vi "control 2.vi"() -> ()   [LabVIEW 2010]
uses:
  <vilib>/Analysis/NI_AALBase.lvlib
panel:
  in  "Ajuste ON?":bool=TRUE
  in  "Control ON?":bool=TRUE
  in  "N Prom":i32
  in  "N Prom inicial":i32
  in  "dSigma":dbl
  in  "dAmp":dbl
  in  "dt0":dbl
  in  "SigmaMax":dbl
  in  "time (ms)":dbl
  in  "# samples":i32
  in  "AmpMax":dbl
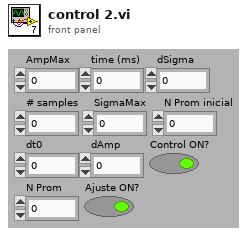
[diagram p1: front panel]
types:
  T1 = cluster{"Amplitud":dbl, "Media":dbl, "Sigma":dbl}
  T2 = cluster{"Amplitud":bool, "Media":bool, "Sigma":bool}
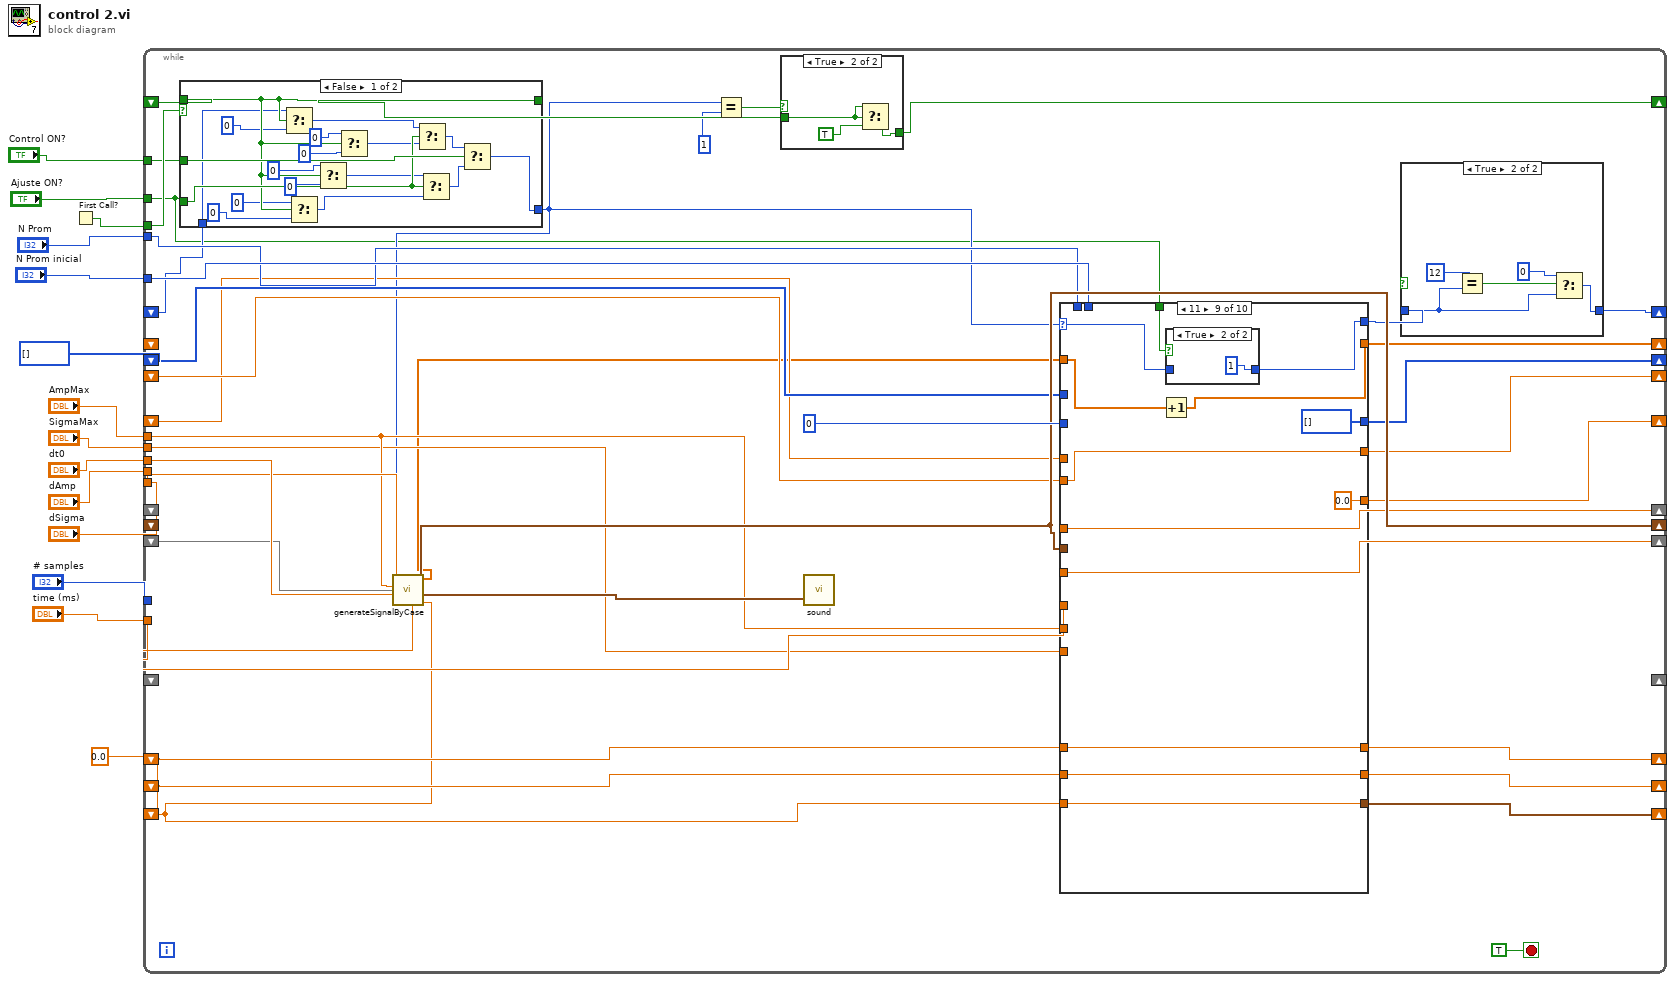
[diagram p0: block diagram]
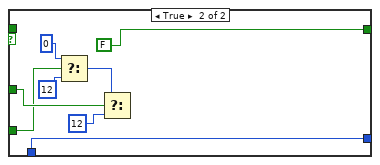
[diagram p3: hidden frame]
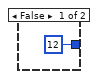
[diagram p4: hidden frame]
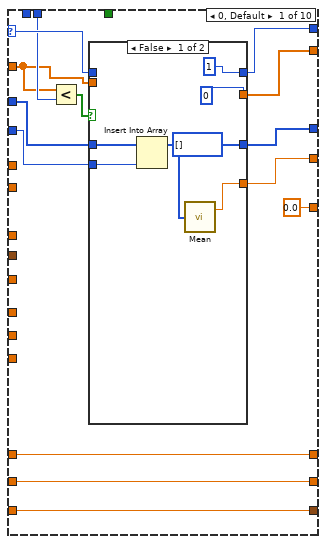
[diagram p5: hidden frame]
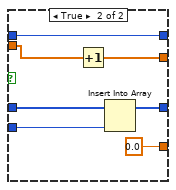
[diagram p6: hidden frame]
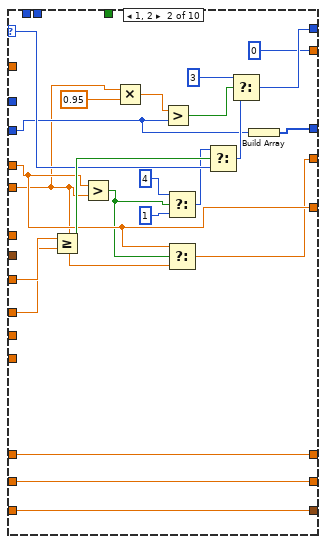
[diagram p7: hidden frame]
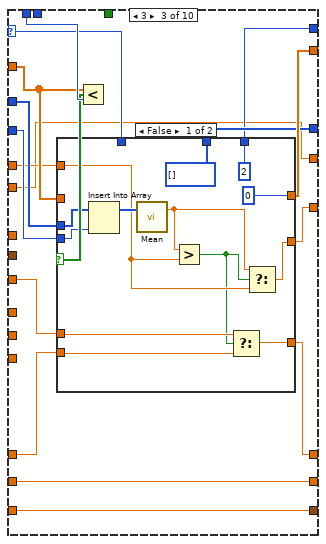
[diagram p8: hidden frame]
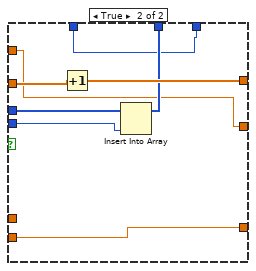
[diagram p9: hidden frame]
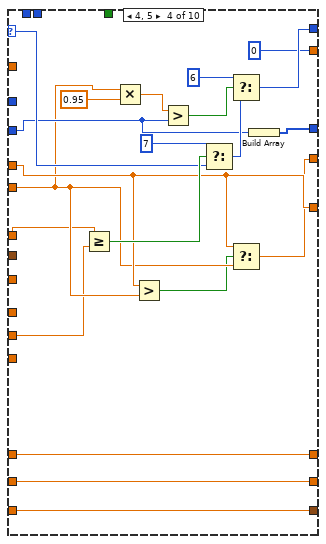
[diagram p10: hidden frame]
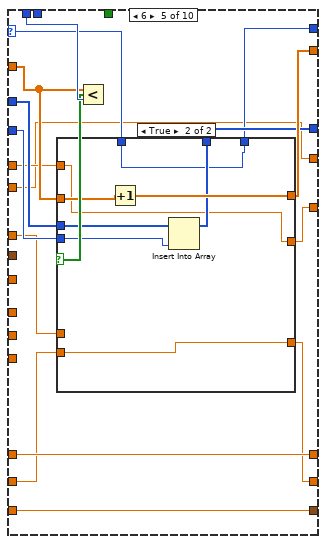
[diagram p11: hidden frame]
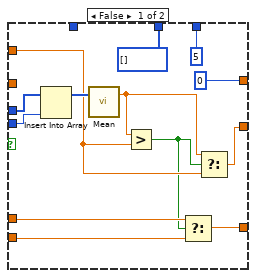
[diagram p12: hidden frame]
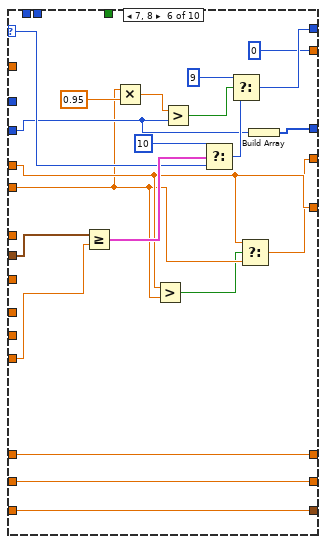
[diagram p13: hidden frame]
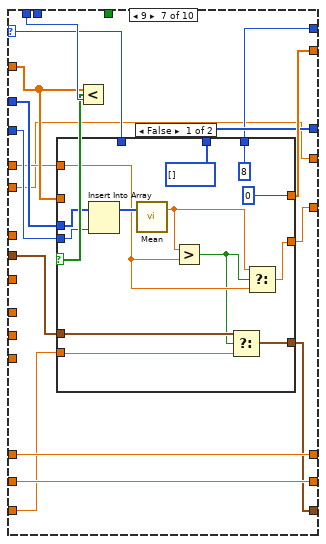
[diagram p14: hidden frame]
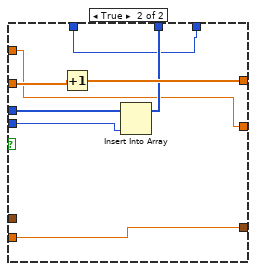
[diagram p15: hidden frame]
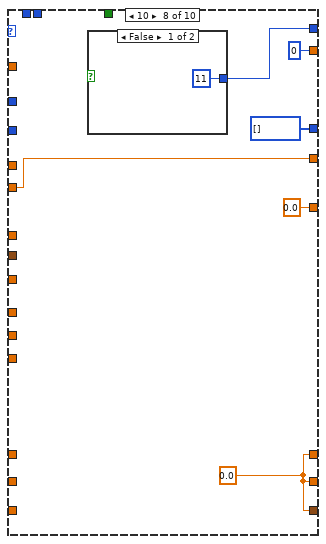
[diagram p16: hidden frame]
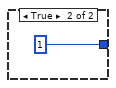
[diagram p17: hidden frame]
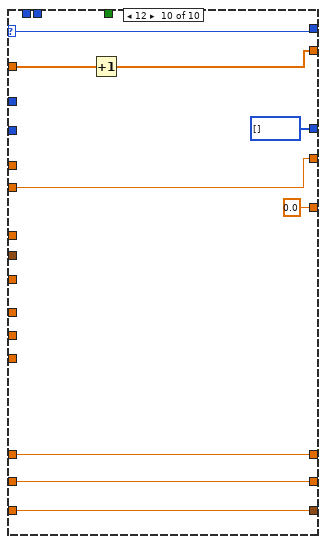
[diagram p19: hidden frame]
diagram:
  w7 = 0.0
  n1 = First Call?() -> (First Call?: T/F=w2:bool)
  n2 = while {
    shift-right: [w56] -> _
    shift-left: _ -> [w52]
    shift-right: [w57] -> _
    shift-left: _ -> [w53]
    shift-right: [w58] -> _
    shift-left: _ -> [w54]
    tunnel: "# samples" -> [w59]
    tunnel: "time (ms)" -> [w41]
    tunnel: "AmpMax" -> [w31]
    tunnel: "SigmaMax" -> [w30]
    tunnel: "dt0" -> [w55]
    shift-right: _ -> [w50]
    shift-left: _ -> [w51]
    shift-right: [w38] -> _
    shift-left: w7 -> [w39]
    shift-right: [w36] -> _
    shift-left: w7 -> [w37]
    tunnel: "dAmp" -> [w49]
    tunnel: "dSigma" -> [w48]
    shift-right: [w34] -> _
    shift-left: w7 -> [w35]
    shift-right: [w26] -> _
    shift-left: _ -> [w17]
    shift-right: [w40] -> _
    shift-left: _ -> [w28]
    shift-right: [w47] -> _
    shift-left: i32[] [] -> [w43]
    tunnel: "N Prom inicial" -> [w46]
    shift-right: [w45] -> _
    shift-left: _ -> [w44]
    tunnel: "N Prom" -> [w42]
    shift-right: [w33] -> _
    shift-left: _ -> [w32]
    tunnel: "Control ON?" -> [w18]
    shift-right: [w21] -> _
    shift-left: _ -> [w23]
    tunnel: w2 -> [w24]
    tunnel: "Ajuste ON?" -> [w15]
    stop <- TRUE stop-if-true
    n3 = case shown="False" w24 {
      tunnel: [w75 FALSE] -> w22
      tunnel: w23 -> [w75 _]
      tunnel: w18 -> [w83 w89]
      tunnel: w15 -> [w80 w88]
      tunnel: w17 -> [w66 w84]
      tunnel: [w74 w84] -> w16
      frame False {
        n4 = Select(t=w66, s=w75, f=u32 0 ("t")) -> (s? t:f=w76:u32)
        n5 = Select(t=u32 0, s=w75, f=u32 0 ("t")) -> (s? t:f=w79:u32)
        n6 = Select(t=u32 0, s=w75, f=u32 0 ("t")) -> (s? t:f=w78:u32)
        n7 = Select(t=u32 0, s=w75, f=u32 0 ("t")) -> (s? t:f=w77:u32)
        n8 = Select(t=w76, s=w80, f=w77) -> (s? t:f=w82:u32)
        n9 = Select(t=w78, s=w80, f=w79) -> (s? t:f=w81:u32)
        n10 = Select(t=w82, s=w83, f=w81) -> (s? t:f=w74:u32)
      }
      frame True {
        n11 = Select(t=u32 0, s=w88, f=u32 12) -> (s? t:f=w90:u32)
        n12 = Select(t=w90, s=w89, f=u32 12) -> ()  [unwired: 1 out]
      }
    }
    n13 = call "generateSignalByCase.vi"("Parametros Iniciales"=w35, "Arreglo de Salida"=w41, "Reset Control"=w54, "detla Parametros"=w48, "Parametros Maximos"=w55, "Sound Parameters"=w31, "ControlCase"=w16) -> ("Mejores Parametros"=w60:T1, "Parametros Actuales"=w57:T1, "Señal de Control OUT"=w27:dbl[])
    n14 = Equal?(x=w16, y=u32 1) -> (x = y?=w19:bool)
    n15 = case shown="True" w19 {
      tunnel: w22 -> [w62 w63]
      tunnel: [w62 w65] -> w21
      frame False {
      }
      frame True {
        n16 = Select(t=w63, s=w63, f=TRUE) -> (s? t:f=w65:bool)
      }
    }
    n17 = call "sound.vi"("df Array"=w60) -> ()  [unwired: 17 in, 2 out]
    n18 = case shown="11" w16 {
      selector: w16 -> [w107 w142 w151 w201 w214 w260 w274 _ w314 w334]
      tunnel: [w108 w144 w150 w203 w213 w262 w273 w305 w315 w334] -> w25
      tunnel: w27 -> [w103 _ w163 _ w222 _ w281 _ w318 w333]
      tunnel: 0 -> [w111 w138 w161 w197 w220 w256 w279 _ _ _]
      tunnel: [w110 w139 w159 w198 w218 w257 w277 i32[] [] i32[] [] i32[] []] -> w47
      tunnel: w43 -> [w109 _ w160 _ w219 _ w278 _ _ _]
      tunnel: w46 -> [w106 _ _ _ _ _ _ _ _ _]
      tunnel: [w104 w128 w149 w190 w212 w249 w272 w309 w323 w330] -> w45
      tunnel: w44 -> [_ w130 w149 w192 w212 w251 w272 w309 w323 w330]
      tunnel: [_ _ _ w187 w208 _ _ _ _ _] -> w56
      tunnel: w57 -> [_ _ _ _ _ w247 w267 _ _ _]
      tunnel: [_ w127 w154 _ _ _ _ _ _ _] -> w58
      tunnel: w42 -> [_ _ w165 _ w224 _ w283 _ _ _]
      tunnel: w41 -> [_ w126 _ _ _ _ _ _ _ _]
      tunnel: [w102 0 w162 0 w221 0 w280 0 w317 w332] -> w40
      tunnel: w39 -> [w101 w137 w153 w196 w211 w255 w271 _ w321 w328]
      tunnel: w37 -> [w100 w136 w158 w195 w210 w254 w270 _ w320 w327]
      tunnel: w35 -> [w99 w135 w157 w194 w217 w253 w269 _ w319 w326]
      tunnel: [w101 w137 w152 w196 w211 w255 w271 w307 w321 w328] -> w38
      tunnel: [w100 w136 w158 w195 w209 w254 w270 w307 w320 w327] -> w36
      tunnel: [w99 w135 w157 w194 w217 w253 w268 w307 w319 w326] -> w34
      tunnel: [0.0 ("mean") w131 w156 w193 w216 w252 w276 0.0 ("mean") 0.0 ("mean") 0.0 ("mean")] -> w33
      tunnel: w32 -> [_ w131 w155 w193 w215 w252 w275 _ _ _]
      tunnel: w31 -> [_ _ _ w188 _ _ _ _ _ _]
      tunnel: w30 -> [_ _ _ _ _ w246 _ _ _ _]
      tunnel: w15 -> [_ _ _ _ _ _ _ _ w313 _]
      frame 0, Default {
        n19 = Less?(x=w103, y=w106) -> (x < y?=w105:bool[])
        n20 = case shown="False" w105 {
          tunnel: w111 -> [w116 w125]
          tunnel: [i32[] [] w124] -> w110
          tunnel: w109 -> [w117 w123]
          tunnel: [1 w122] -> w108
          tunnel: w107 -> [_ w122]
          tunnel: [w113 0.0 ("mean")] -> w104
          tunnel: w103 -> [_ w120]
          tunnel: [0 w119] -> w102
          frame False {
            n21 = Insert Into Array(array=w117, new element=w116) -> (w115:i32[])  [unwired: 1 in]
            n22 = call <vilib>:"Mean.vi"("X"=w115) -> ("mean"=w113:dbl)  [unwired: 1 out]
          }
          frame True {
            n23 = Increment(x=w120) -> (x+1=w119:dbl[])
            n24 = Insert Into Array(array=w123, new element=w125) -> (w124:i32[])  [unwired: 1 in]
          }
        }
      }
      frame 1, 2 {
        n25 = Greater Or Equal?(x=w127, y=w126) -> (x >= y?=w143:bool)
        n26 = Greater?(x=w131, y=w130) -> (0:w129:bool)
        n27 = Multiply(x=w130, y=0.95) -> (x*y=w147:dbl)
        n28 = Greater?(x=w147, y=w138) -> (0:w146:bool)
        n29 = Select(t=u32 4, s=w129, f=u32 1) -> (s? t:f=w134:u32)
        n30 = Select(t=w131, s=w129, f=w130) -> (s? t:f=w128:dbl)
        n31 = Select(t=w134, s=w143, f=w142) -> (s? t:f=w141:u32)
        n32 = Select(t=u32 3, s=w146, f=w141) -> (s? t:f=w144:u32)
        n33 = Build Array(w138) -> (w139:i32[])
      }
      frame 3 {
        n34 = Less?(x=w163, y=w165) -> (x < y?=w164:bool[])
        n35 = case shown="False" w164 {
          tunnel: w163 -> [_ w186]
          tunnel: [0 w185] -> w162
          tunnel: w161 -> [w178 w183]
          tunnel: w160 -> [w177 w184]
          tunnel: [i32[] [] w182] -> w159
          tunnel: [w172 w180] -> w156
          tunnel: w155 -> [w169 w180]
          tunnel: w154 -> [w171 _]
          tunnel: w153 -> [w170 w179]
          tunnel: [w167 w179] -> w152
          tunnel: w151 -> [_ w181]
          tunnel: [u32 2 ("t") w181] -> w150
          frame False {
            n36 = Insert Into Array(array=w177, new element=w178) -> (w176:i32[])  [unwired: 1 in]
            n37 = call <vilib>:"Mean.vi"("X"=w176) -> ("mean"=w173:dbl)  [unwired: 1 out]
            n38 = Greater?(x=w173, y=w169) -> (0:w168:bool)
            n39 = Select(t=w171, s=w168, f=w170) -> (s? t:f=w167:dbl)
            n40 = Select(t=w173, s=w168, f=w169) -> (s? t:f=w172:dbl)
          }
          frame True {
            n41 = Increment(x=w186) -> (x+1=w185:dbl[])
            n42 = Insert Into Array(array=w184, new element=w183) -> (w182:i32[])  [unwired: 1 in]
          }
        }
      }
      frame 4, 5 {
        n43 = Greater Or Equal?(x=w187, y=w188) -> (x >= y?=w202:bool)
        n44 = Multiply(x=w192, y=0.95) -> (x*y=w206:dbl)
        n45 = Greater?(x=w193, y=w192) -> (0:w191:bool)
        n46 = Greater?(x=w206, y=w197) -> (0:w205:bool)
        n47 = Select(t=u32 7, s=w202, f=w201) -> (s? t:f=w200:u32)
        n48 = Select(t=u32 6, s=w205, f=w200) -> (s? t:f=w203:u32)
        n49 = Select(t=w193, s=w191, f=w192) -> (s? t:f=w190:dbl)
        n50 = Build Array(w197) -> (w198:i32[])
      }
      frame 6 {
        n51 = Less?(x=w222, y=w224) -> (x < y?=w223:bool[])
        n52 = case shown="True" w223 {
          tunnel: w222 -> [_ w245]
          tunnel: [0 w244] -> w221
          tunnel: w220 -> [w237 w242]
          tunnel: w219 -> [w236 w243]
          tunnel: [i32[] [] w241] -> w218
          tunnel: [w231 w239] -> w216
          tunnel: w215 -> [w228 w239]
          tunnel: w208 -> [w230 _]
          tunnel: w210 -> [w229 w238]
          tunnel: [w226 w238] -> w209
          tunnel: w214 -> [_ w240]
          tunnel: [u32 5 ("t") w240] -> w213
          frame False {
            n53 = Insert Into Array(array=w236, new element=w237) -> (w235:i32[])  [unwired: 1 in]
            n54 = call <vilib>:"Mean.vi"("X"=w235) -> ("mean"=w232:dbl)  [unwired: 1 out]
            n55 = Greater?(x=w232, y=w228) -> (0:w227:bool)
            n56 = Select(t=w230, s=w227, f=w229) -> (s? t:f=w226:dbl)
            n57 = Select(t=w232, s=w227, f=w228) -> (s? t:f=w231:dbl)
          }
          frame True {
            n58 = Increment(x=w245) -> (x+1=w244:dbl[])
            n59 = Insert Into Array(array=w243, new element=w242) -> (w241:i32[])  [unwired: 1 in]
          }
        }
      }
      frame 7, 8 {
        n60 = Greater Or Equal?(x=w247, y=w246) -> (x >= y?=w261:T2)
        n61 = Multiply(x=w251, y=0.95) -> (x*y=w265:dbl)
        n62 = Greater?(x=w252, y=w251) -> (0:w250:bool)
        n63 = Greater?(x=w265, y=w256) -> (0:w264:bool)
        n64 = Select(t=u32 10, s=w261, f=w260) -> (s? t:f=w259:u32)
        n65 = Select(t=u32 9, s=w264, f=w259) -> (s? t:f=w262:u32)
        n66 = Select(t=w252, s=w250, f=w251) -> (s? t:f=w249:dbl)
        n67 = Build Array(w256) -> (w257:i32[])
      }
      frame 9 {
        n68 = Less?(x=w281, y=w283) -> (x < y?=w282:bool[])
        n69 = case shown="False" w282 {
          tunnel: w281 -> [_ w304]
          tunnel: [0 w303] -> w280
          tunnel: w279 -> [w296 w301]
          tunnel: w278 -> [w295 w302]
          tunnel: [i32[] [] w300] -> w277
          tunnel: [w290 w298] -> w276
          tunnel: w275 -> [w287 w298]
          tunnel: w267 -> [w289 _]
          tunnel: w269 -> [w288 w297]
          tunnel: [w285 w297] -> w268
          tunnel: w274 -> [_ w299]
          tunnel: [u32 8 ("t") w299] -> w273
          frame False {
            n70 = Insert Into Array(array=w295, new element=w296) -> (w294:i32[])  [unwired: 1 in]
            n71 = call <vilib>:"Mean.vi"("X"=w294) -> ("mean"=w291:dbl)  [unwired: 1 out]
            n72 = Greater?(x=w291, y=w287) -> (0:w286:bool)
            n73 = Select(t=w289, s=w286, f=w288) -> (s? t:f=w285:T1)
            n74 = Select(t=w291, s=w286, f=w287) -> (s? t:f=w290:dbl)
          }
          frame True {
            n75 = Increment(x=w304) -> (x+1=w303:dbl[])
            n76 = Insert Into Array(array=w302, new element=w301) -> (w300:i32[])  [unwired: 1 in]
          }
        }
      }
      frame 10 {
        w307 = 0.0
        n77 = case shown="False" {
          selector: _ -> [_ _]
          tunnel: [u32 11 ("t") u32 1 ("t")] -> w305
          frame False {
          }
          frame True {
          }
        }
      }
      frame 11 {
        n78 = Increment(x=w318) -> (x+1=w317:dbl[])
        n79 = case shown="True" w313 {
          tunnel: [w324 1] -> w315
          tunnel: w314 -> [w324 _]
          frame False {
          }
          frame True {
          }
        }
      }
      frame 12 {
        n80 = Increment(x=w333) -> (x+1=w332:dbl[])
      }
    }
    n81 = case shown="True" {
      selector: _ -> [_ _]
      tunnel: [u32 12 ("t") w93] -> w26
      tunnel: w25 -> [_ w95]
      frame False {
      }
      frame True {
        n82 = Equal?(x=u32 12, y=w95) -> (x = y?=w96:bool)
        n83 = Select(t=u32 0, s=w96, f=w95) -> (s? t:f=w93:u32)
      }
    }
  }
